vi "Get Strain Log File.vi"(8 "error in (no error)":errorcluster, 10 "Time Stamp":timestamp, 11 "Strain Logger in":refnum<class "Strain Logger.lvclass">) -> (0 "error out":errorcluster, 2 "Log file name":path=path "C:/Data", 3 "Strain Logger out":refnum<class "Strain Logger.lvclass">)   [LabVIEW 2024, in "Strain Logger.lvclass"]
uses:
  Strain Logger.lvclass
  Strain Logger.lvclass/Strain Logger.ctl
panel:
  in  "Root Data Folder":path=path "C:/Data"
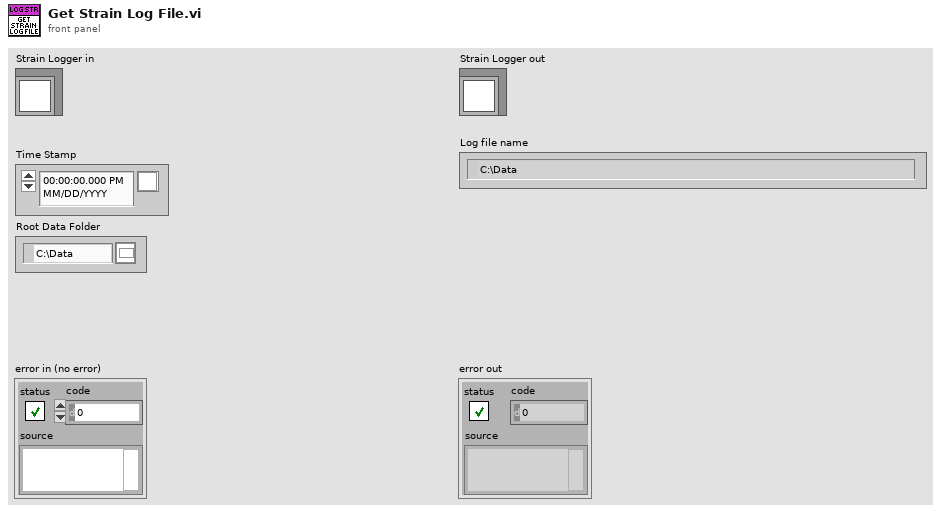
[diagram p1: front panel]
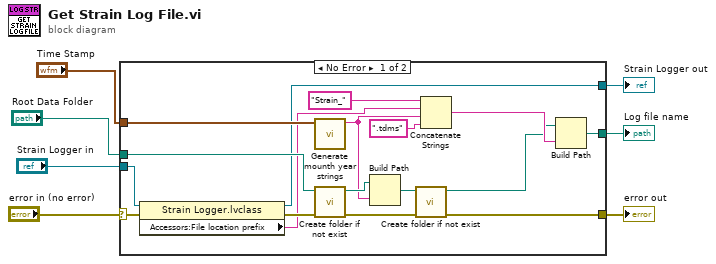
[diagram p0: block diagram]
diagram:
  n1 = case shown="No Error" "error in (no error)" {
    selector: "error in (no error)" -> [w20 w26]
    tunnel: [w8 w26] -> w6
    tunnel: [w12 w25] -> w4
    tunnel: "Strain Logger in" -> [w13 w25]
    tunnel: "Root Data Folder" -> [w24 _]
    tunnel: "Time Stamp" -> [w22 _]
    tunnel: [w15 _] -> w1
    frame No Error {
      n2 = property class="Strain Logger.lvclass"(reference=w13, error in=w20) -> (reference out=w12:refnum<class "Strain Logger.lvclass">, error out=w14:errorcluster, "Accessors:File location prefix"=w10:string)
      n3 = call "Generate mounth year strings.vi"("Time Stamp (default 0 = now)"=w22) -> ("Month_year"=w18:string)  [unwired: 1 in, 9 out]
      n4 = call "Create folder if not exist.vi"("Error In"=w14, "Folder Path Control"=w24) -> ("Error Out"=w19:errorcluster, "Folder Path out"=w23:path)  [unwired: 8 out]
      n5 = Build Path(base path=w23, name or relative path=w18) -> (appended path=w21:path)
      n6 = call "Create folder if not exist.vi"("Error In"=w19, "Folder Path Control"=w21) -> ("Error Out"=w8:errorcluster, "Folder Path out"=w9:path)  [unwired: 8 out]
      n7 = Concatenate Strings("Strain_" ("string"), w10, w18, ".tdms" ("string")) -> (w16:string)
      n8 = Build Path(base path=w9, name or relative path=w16) -> (appended path=w15:path)
    }
    frame Error {
    }
  }
  "error out" <- w6
  "Strain Logger out" <- w4
  "Log file name" <- w1
